vi "(Instrl) HVPS_1.vi"(1 "Write Data":string, 2 "IP":string, 3 "Port":u16, 5 "error in (no error)":errorcluster caption="에러 입력(에러 없음)", 6 "CMD":T1=enum."Rx : V") -> (14 "Get V":dbl, 15 "Get mA":dbl, 16 "System State":string, 17 "HV State":string, 18 "Operation Mode":string, 19 "error out":errorcluster caption="에러 출력")   [LabVIEW 2017]
uses:
  Controls/(Ctrl) State_HVPS CMD.ctl
  Controls/(Ctrl) State_Write CMD.ctl
  Controls/(Ctrl) State_Parcing.ctl
panel:
  out "Read":string
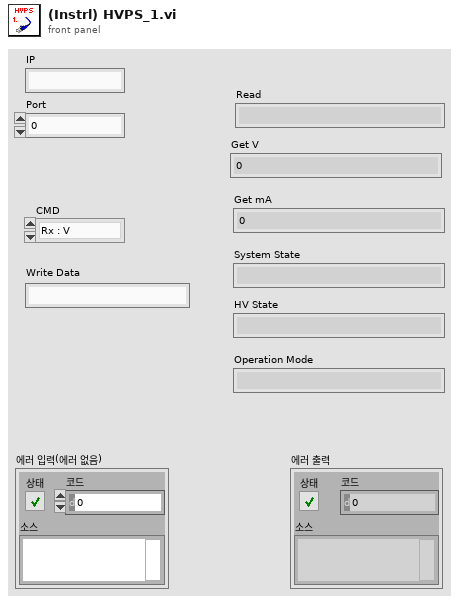
[diagram p1: front panel]
types:
  T1 = typedef "(Ctrl) State_HVPS CMD.ctl" = enum16{"Open", "Rx : V", "Rx : mA", "Rx : State", "Rx : ADC", "Tx : Set V", "Tx : Set mA", "Tx : ON", "Tx : OFF", "Close"}
  T2 = typedef "(Ctrl) State_Parcing.ctl" = enum16{"Default", "Set V", "Set mA", "Get V", "Get mA", "Get ADC"}
  T3 = enum16{"Standard", "Buffered", "CRLF", "Immediate"}
  T4 = typedef "(Ctrl) State_Write CMD.ctl" = enum16{"Defalut", "Set KV", "Set mA", "Get KV", "Get mA", "Get ADC", "HV On", "HV Off", "System State", "HV State", "Opration Mode"}
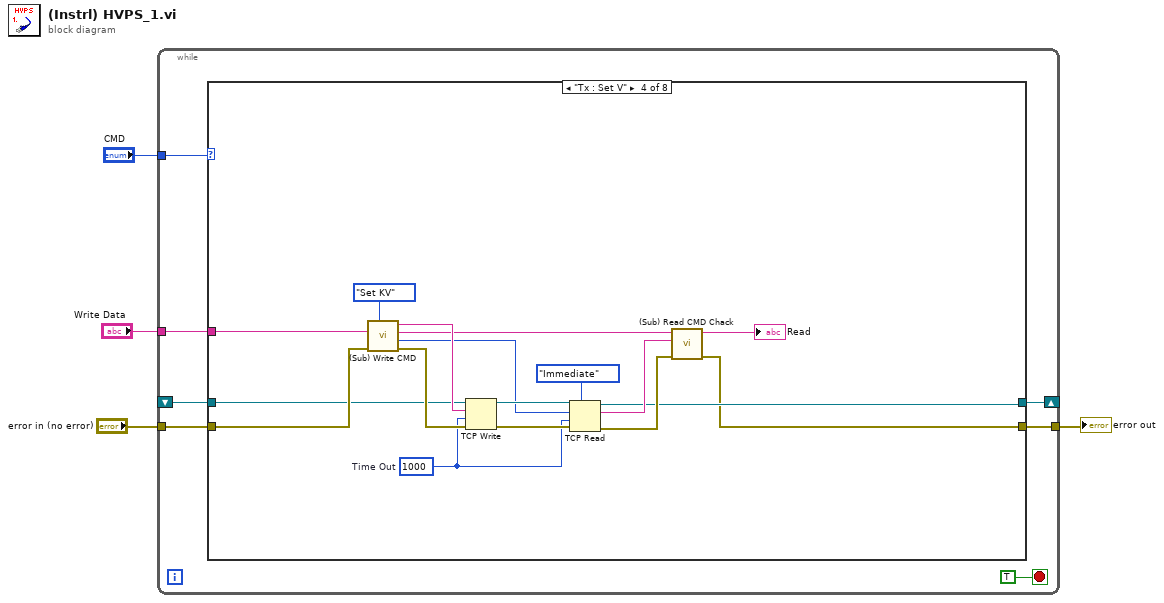
[diagram p0: block diagram]
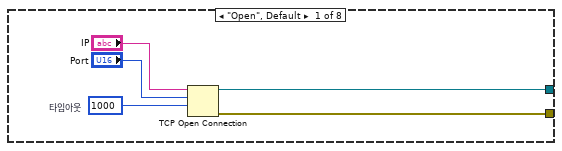
[diagram p2: hidden frame]
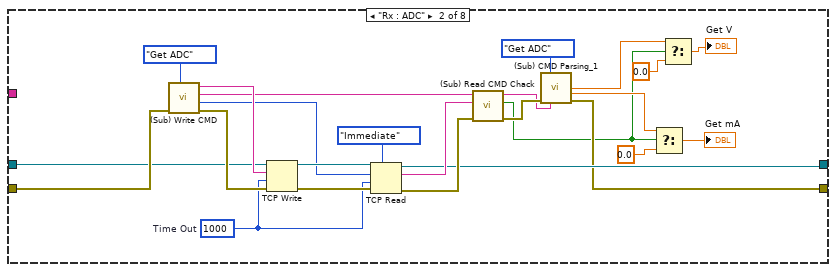
[diagram p3: hidden frame]
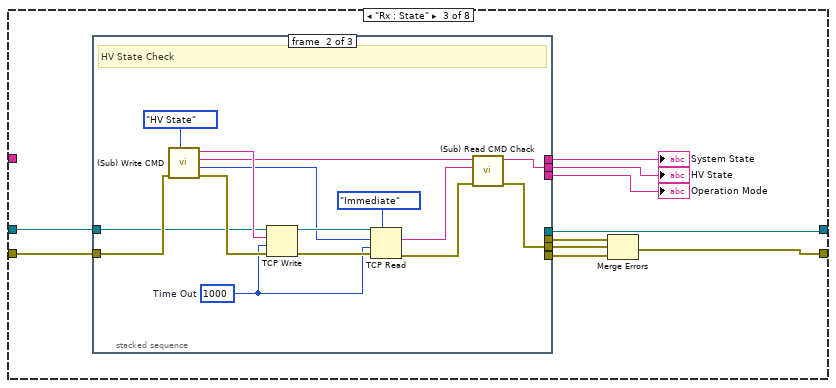
[diagram p4: hidden frame]
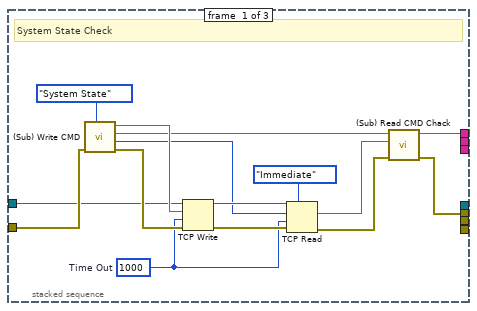
[diagram p5: hidden frame]
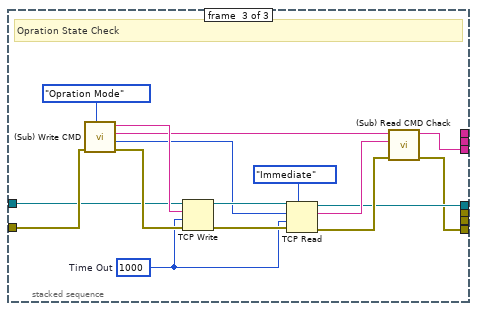
[diagram p6: hidden frame]
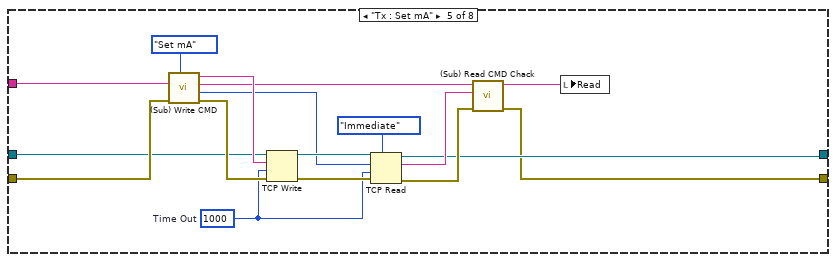
[diagram p7: hidden frame]
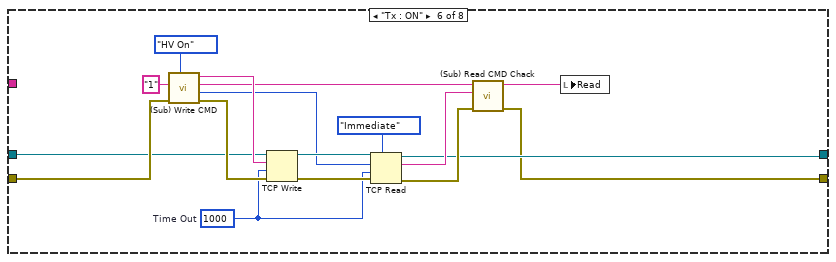
[diagram p8: hidden frame]
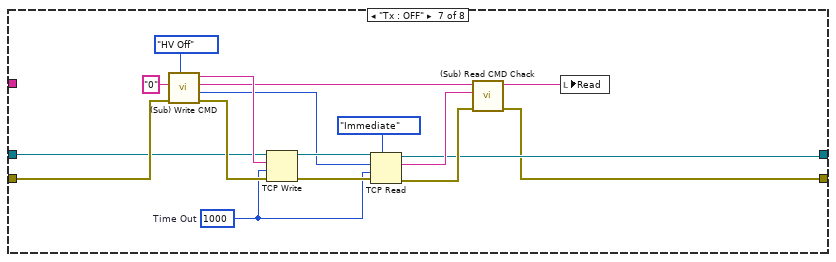
[diagram p9: hidden frame]
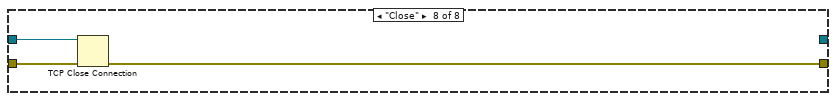
[diagram p10: hidden frame]
diagram:
  n1 = while {
    tunnel: "CMD" -> [w9]
    tunnel: "Write Data" -> [w8]
    shift-right: [w6] -> _
    shift-left: _ -> [w7]
    tunnel: "error in (no error)" -> [w11]
    tunnel: [w10] -> w3
    stop <- TRUE stop-if-true
    n2 = case shown="\"Tx : Set V\"" w9 {
      tunnel: [w16 w28 w49 w101 w118 w135 w152 _] -> w6
      tunnel: [w15 w26 w42 w99 w116 w134 w151 w166] -> w10
      tunnel: w11 -> [_ w40 w51 w113 w130 w147 w164 w167]
      tunnel: w7 -> [_ w37 w50 w110 w127 w144 w161 w168]
      tunnel: w8 -> [_ _ _ w100 w117 _ _ _]
      frame "Open", Default {
        w12 = 1000  # 타임아웃
        n3 = TCP Open Connection ("TCP 연결 열기")(address="IP", remote port or service name="Port", timeout ms (60000)=w12) -> (connection ID=w16:refnum<k5>, error out=w15:errorcluster)  [unwired: 2 in]
      }
      frame "Rx : ADC" {
        w35 = 1000  # Time Out
        n4 = call "(Sub) Write CMD.vi"("State"=(Ctrl)_State_Write_CMD."Get ADC", "error in (no error)"=w40) -> ("error out"=w39:errorcluster, "Read Byte"=w32:i32, "CMD"=w29:string, "Write CMD"=w38:string)  [unwired: 6 in]
        n5 = TCP Write ("TCP 쓰기")(connection ID=w37, data in=w38, error in (no error)=w39, 9:w35) -> (connection ID out=w34:refnum<k5>, error out=w36:errorcluster)  [unwired: 1 out]
        n6 = TCP Read ("TCP 읽기")(connection ID=w34, bytes to read=w32, error in (no error)=w36, 7:T3."Immediate" ("모드(standard)"), 9:w35) -> (connection ID out=w28:refnum<k5>, data out=w30:string, error out=w31:errorcluster)
        n7 = call "(Sub) Read CMD Chack.vi"("error in (no error)"=w31, "Read Data"=w30, "Write CMD"=w29) -> ("error out"=w27:errorcluster, "Read Success ?"=w19:bool, "Data"=w22:string)  [unwired: 6 in]
        n8 = call "(Sub) CMD Parsing_1.vi"("State"=(Ctrl)_State_Parcing."Get ADC", "error in (no error)"=w27, "CMD Get ADC"=w22) -> ("Get KV"=w21:dbl, "Get mA"=w24:dbl, "error out"=w26:errorcluster)  [unwired: 8 in, 2 out]
        n9 = Select(t=w24, s=w19, f=0.0) -> (s? t:f=→"Get mA":dbl)
        n10 = Select(t=w21, s=w19, f=0.0) -> (s? t:f=→"Get V":dbl)
      }
      frame "Rx : State" {
        n11 = stacked-sequence {
          tunnel: w51 -> [w65 w80 w96]
          tunnel: w50 -> [w62 w77 w93]
          tunnel: [_ _ w84] -> w49
          tunnel: [w53 _ _] -> w48
          tunnel: [_ w68 _] -> w47
          tunnel: [_ _ w83] -> w46
          tunnel: [_ _ w82] -> w43
          tunnel: [w52 _ _] -> w45
          tunnel: [_ w67 _] -> w44
          frame #0 {
            w60 = 1000  # Time Out
            # "System State Check"
            n12 = call "(Sub) Write CMD.vi"("State"=(Ctrl)_State_Write_CMD."System State", "error in (no error)"=w65) -> ("error out"=w64:errorcluster, "Read Byte"=w57:i32, "CMD"=w54:string, "Write CMD"=w63:string)  [unwired: 6 in]
            n13 = TCP Write ("TCP 쓰기")(connection ID=w62, data in=w63, error in (no error)=w64, 9:w60) -> (connection ID out=w59:refnum<k5>, error out=w61:errorcluster)  [unwired: 1 out]
            n14 = TCP Read ("TCP 읽기")(connection ID=w59, bytes to read=w57, error in (no error)=w61, 7:T3."Immediate" ("모드(standard)"), 9:w60) -> (data out=w55:string, error out=w56:errorcluster)  [unwired: 1 out]
            n15 = call "(Sub) Read CMD Chack.vi"("error in (no error)"=w56, "Read Data"=w55, "Write CMD"=w54) -> ("error out"=w52:errorcluster, "Data"=w53:string)  [unwired: 6 in, 1 out]
          }
          frame #1 {
            w75 = 1000  # Time Out
            # "HV State Check"
            n16 = call "(Sub) Write CMD.vi"("State"=(Ctrl)_State_Write_CMD."HV State", "error in (no error)"=w80) -> ("error out"=w79:errorcluster, "Read Byte"=w72:i32, "CMD"=w69:string, "Write CMD"=w78:string)  [unwired: 6 in]
            n17 = TCP Write ("TCP 쓰기")(connection ID=w77, data in=w78, error in (no error)=w79, 9:w75) -> (connection ID out=w74:refnum<k5>, error out=w76:errorcluster)  [unwired: 1 out]
            n18 = TCP Read ("TCP 읽기")(connection ID=w74, bytes to read=w72, error in (no error)=w76, 7:T3."Immediate" ("모드(standard)"), 9:w75) -> (data out=w70:string, error out=w71:errorcluster)  [unwired: 1 out]
            n19 = call "(Sub) Read CMD Chack.vi"("error in (no error)"=w71, "Read Data"=w70, "Write CMD"=w69) -> ("error out"=w67:errorcluster, "Data"=w68:string)  [unwired: 6 in, 1 out]
          }
          frame #2 {
            w91 = 1000  # Time Out
            # "Opration State Check"
            n20 = call "(Sub) Write CMD.vi"("State"=(Ctrl)_State_Write_CMD."Opration Mode", "error in (no error)"=w96) -> ("error out"=w95:errorcluster, "Read Byte"=w88:i32, "CMD"=w85:string, "Write CMD"=w94:string)  [unwired: 6 in]
            n21 = TCP Write ("TCP 쓰기")(connection ID=w93, data in=w94, error in (no error)=w95, 9:w91) -> (connection ID out=w90:refnum<k5>, error out=w92:errorcluster)  [unwired: 1 out]
            n22 = TCP Read ("TCP 읽기")(connection ID=w90, bytes to read=w88, error in (no error)=w92, 7:T3."Immediate" ("모드(standard)"), 9:w91) -> (connection ID out=w84:refnum<k5>, data out=w86:string, error out=w87:errorcluster)
            n23 = call "(Sub) Read CMD Chack.vi"("error in (no error)"=w87, "Read Data"=w86, "Write CMD"=w85) -> ("error out"=w82:errorcluster, "Data"=w83:string)  [unwired: 6 in, 1 out]
          }
        }
        "System State" <- w48
        "HV State" <- w47
        "Operation Mode" <- w46
        n24 = Merge Errors(w45, w44, w43) -> (w42:errorcluster)
      }
      frame "Tx : Set V" {
        w108 = 1000  # Time Out
        n25 = call "(Sub) Write CMD.vi"("State"=(Ctrl)_State_Write_CMD."Set KV", "error in (no error)"=w113, "Write Data"=w100) -> ("error out"=w112:errorcluster, "Read Byte"=w105:i32, "CMD"=w102:string, "Write CMD"=w111:string)  [unwired: 5 in]
        n26 = TCP Write ("TCP 쓰기")(connection ID=w110, data in=w111, error in (no error)=w112, 9:w108) -> (connection ID out=w107:refnum<k5>, error out=w109:errorcluster)  [unwired: 1 out]
        n27 = TCP Read ("TCP 읽기")(connection ID=w107, bytes to read=w105, error in (no error)=w109, 7:T3."Immediate" ("모드(standard)"), 9:w108) -> (connection ID out=w101:refnum<k5>, data out=w103:string, error out=w104:errorcluster)
        n28 = call "(Sub) Read CMD Chack.vi"("error in (no error)"=w104, "Read Data"=w103, "Write CMD"=w102) -> ("error out"=w99:errorcluster, "Data"=→"Read":string)  [unwired: 6 in, 1 out]
      }
      frame "Tx : Set mA" {
        w125 = 1000  # Time Out
        n29 = call "(Sub) Write CMD.vi"("State"=(Ctrl)_State_Write_CMD."Set mA", "error in (no error)"=w130, "Write Data"=w117) -> ("error out"=w129:errorcluster, "Read Byte"=w122:i32, "CMD"=w119:string, "Write CMD"=w128:string)  [unwired: 5 in]
        n30 = TCP Write ("TCP 쓰기")(connection ID=w127, data in=w128, error in (no error)=w129, 9:w125) -> (connection ID out=w124:refnum<k5>, error out=w126:errorcluster)  [unwired: 1 out]
        n31 = TCP Read ("TCP 읽기")(connection ID=w124, bytes to read=w122, error in (no error)=w126, 7:T3."Immediate" ("모드(standard)"), 9:w125) -> (connection ID out=w118:refnum<k5>, data out=w120:string, error out=w121:errorcluster)
        n32 = call "(Sub) Read CMD Chack.vi"("error in (no error)"=w121, "Read Data"=w120, "Write CMD"=w119) -> ("error out"=w116:errorcluster, "Data"=w115:string)  [unwired: 6 in, 1 out]
        n33 = local write "Read"(w115) -> ()
      }
      frame "Tx : ON" {
        w142 = 1000  # Time Out
        n34 = call "(Sub) Write CMD.vi"("State"=(Ctrl)_State_Write_CMD."HV On", "error in (no error)"=w147, "Write Data"="1") -> ("error out"=w146:errorcluster, "Read Byte"=w139:i32, "CMD"=w136:string, "Write CMD"=w145:string)  [unwired: 5 in]
        n35 = TCP Write ("TCP 쓰기")(connection ID=w144, data in=w145, error in (no error)=w146, 9:w142) -> (connection ID out=w141:refnum<k5>, error out=w143:errorcluster)  [unwired: 1 out]
        n36 = TCP Read ("TCP 읽기")(connection ID=w141, bytes to read=w139, error in (no error)=w143, 7:T3."Immediate" ("모드(standard)"), 9:w142) -> (connection ID out=w135:refnum<k5>, data out=w137:string, error out=w138:errorcluster)
        n37 = call "(Sub) Read CMD Chack.vi"("error in (no error)"=w138, "Read Data"=w137, "Write CMD"=w136) -> ("error out"=w134:errorcluster, "Data"=w133:string)  [unwired: 6 in, 1 out]
        n38 = local write "Read"(w133) -> ()
      }
      frame "Tx : OFF" {
        w159 = 1000  # Time Out
        n39 = call "(Sub) Write CMD.vi"("State"=(Ctrl)_State_Write_CMD."HV Off", "error in (no error)"=w164, "Write Data"="0") -> ("error out"=w163:errorcluster, "Read Byte"=w156:i32, "CMD"=w153:string, "Write CMD"=w162:string)  [unwired: 5 in]
        n40 = TCP Write ("TCP 쓰기")(connection ID=w161, data in=w162, error in (no error)=w163, 9:w159) -> (connection ID out=w158:refnum<k5>, error out=w160:errorcluster)  [unwired: 1 out]
        n41 = TCP Read ("TCP 읽기")(connection ID=w158, bytes to read=w156, error in (no error)=w160, 7:T3."Immediate" ("모드(standard)"), 9:w159) -> (connection ID out=w152:refnum<k5>, data out=w154:string, error out=w155:errorcluster)
        n42 = call "(Sub) Read CMD Chack.vi"("error in (no error)"=w155, "Read Data"=w154, "Write CMD"=w153) -> ("error out"=w151:errorcluster, "Data"=w150:string)  [unwired: 6 in, 1 out]
        n43 = local write "Read"(w150) -> ()
      }
      frame "Close" {
        n44 = TCP Close Connection(connection ID=w168, error in (no error)=w167) -> (error out=w166:errorcluster)  [unwired: 1 in, 1 out]
      }
    }
  }
  "error out" <- w3
